vi "Get Fields.vi"(8 "error in (no error)":errorcluster, 11 "variant":variant) -> (0 "error out":errorcluster, 1 "Types":T1[](array[typedef]), 2 "element variant array":variant[](array[variant]), 3 "Fieldnames":string[](array[string]), 5 "empty variant array":variant[](array[variant]))   [LabVIEW 2019]
uses:
  <vilib>/Utility/Data Type/Type Definitions/Data Type.ctl
  <vilib>/Utility/Data Type/NI_Data Type.lvlib
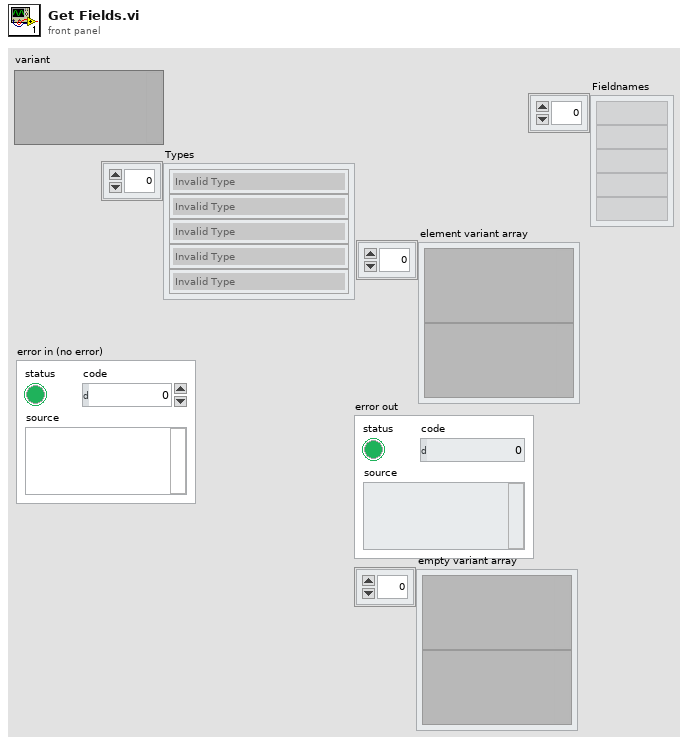
[diagram p1: front panel]
types:
  T1 = typedef "NI_Data Type.lvlib/Data Type.ctl" = enum8{"Invalid Type", "Void", "I8", "I16", "I32", "I64", "U8", "U16", "U32", "U64", "Single Float", "Double Float", "Extended Float", "Single Complex", "Double Complex", "Extended Complex", "Enum U8", "Enum U16", "Enum U32", "Enum U64", "Single Float With Unit", "Double Float With Unit", "Extended Float With Unit", "Single Complex with Unit", "Double Complex with Unit", "Extended Complex with Unit", "Boolean", "String", "Path", "Picture", "Tag", "Array", "Cluster", "Variant", "LV Variant", "Waveform", "Timestamp", "Digital Waveform", "Digital Data", "ExpressData", "Refnum", "External Data", "VI", "Poly VI", "LabVIEW Class Instance", "Fixed Point", "Set Collection", "Map Collection"}
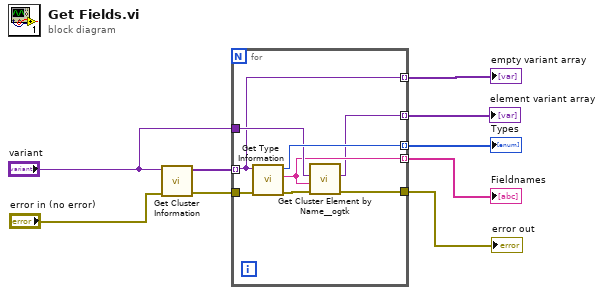
[diagram p0: block diagram]
diagram:
  n1 = call <vilib>:"Get Cluster Information.vi"("error in (no error)"="error in (no error)", "variant"="variant") -> ("error out"=w7:errorcluster, "cluster elements"=w8:variant[])  [unwired: 8 in]
  n2 = for {
    tunnel: w8 -> [w10] mode=indexing
    tunnel: w7 -> [w17]
    tunnel: [w14] -> w6 mode=indexing
    tunnel: [w11] -> w5
    tunnel: [w16] -> w4 mode=indexing
    tunnel: "variant" -> [w15]
    tunnel: [w13] -> w2 mode=indexing
    tunnel: [w10] -> w1 mode=indexing
    n3 = call <vilib>:"Get Type Information.vi"("error in (no error)"=w17, "variant"=w10) -> ("error out"=w12:errorcluster, "name"=w14:string, "type"=w16:T1)  [unwired: 5 in, 2 out]
    n4 = call <userlib>:"Get Cluster Element by Name__ogtk.vi"("error in (no error)"=w12, "Element Name"=w14, "Cluster"=w15) -> ("error out"=w11:errorcluster, "VElement"=w13:variant)  [unwired: 6 in, 1 out]
  }
  "Fieldnames" <- w6
  "error out" <- w5
  "Types" <- w4
  "element variant array" <- w2
  "empty variant array" <- w1
